vi "Write Config Data VI.vi"(8 "error in (no error)":errorcluster, 10 "Config Data":T1={"DS First Launch"=FALSE, "LogBaseFolder"=path "", "Live Logging"=FALSE, "Server Port"=0, "Max Number ML Rows"=0, "AM.WinBounds"={"Left"=0, "Top"=0, "Right"=0, "Bottom"=0}, "AM.FP.State"=enum."Invalid", "AM.Monitor"=0, "AM.Column Widths"=[], "ML.Visible Columns"=[], "ML.Splitter Position"=0, "ML.Column Widths"=[], "ML.WinBounds"={"Left"=0, "Top"=0, "Right"=0, "Bottom"=0}, "ML.FP.State"=enum."Invalid", "ML.Monitor"=0}, 11 "Settings in":refnum<class "Settings.lvclass">) -> (0 "error out":errorcluster, 3 "Settings out":refnum<class "Settings.lvclass">)   [LabVIEW 2017, in "Settings.lvclass"]
uses:
  Settings.lvclass
  Config Data.ctl
  <vilib>/Utility/miscctls.llb/LVRectTypeDef.ctl
  <vilib>/Utility/config.llb/Write Key (Boolean).vi
  <vilib>/Utility/config.llb/Write Key (Path).vi
  <vilib>/Utility/config.llb/Write Key (U32).vi
  <vilib>/Utility/config.llb/Write Key (String).vi
  <vilib>/Utility/config.llb/Write Key (I32).vi
  <vilib>/Utility/config.llb/NI_LVConfig.lvlib
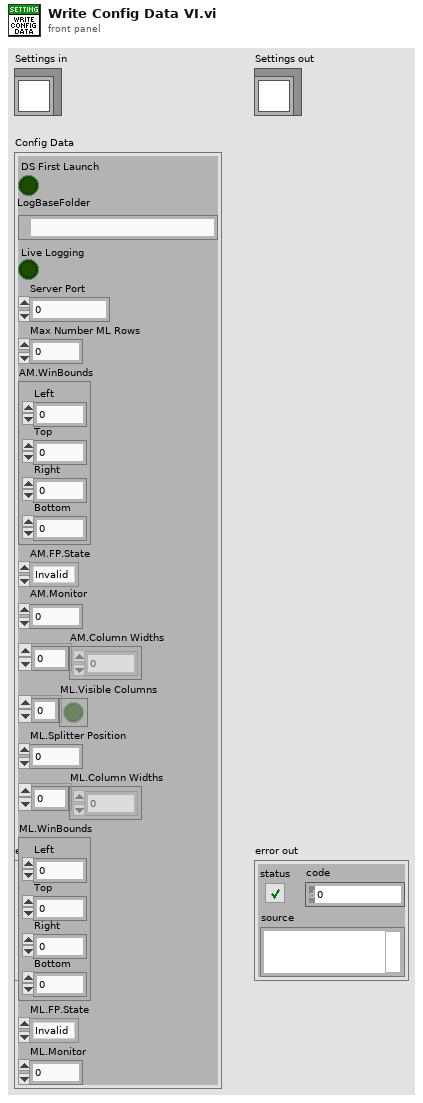
[diagram p1: front panel]
types:
  T1 = typedef "Settings.lvclass/Config Data.ctl" = cluster{"DS First Launch":bool, "LogBaseFolder":path, "Live Logging":bool, "Server Port":u16, "Max Number ML Rows":i32, "AM.WinBounds":T2, "AM.FP.State":enum32{"Invalid", "Standard", "Closed", "Hidden", "Minimized", "Maximized"}, "AM.Monitor":u16, "AM.Column Widths":u32[], "ML.Visible Columns":bool[], "ML.Splitter Position":i32, "ML.Column Widths":u32[], "ML.WinBounds":T2, "ML.FP.State":enum32{"Invalid", "Standard", "Closed", "Hidden", "Minimized", "Maximized"}, "ML.Monitor":u16}
  T2 = typedef "LVRectTypeDef.ctl" = cluster{"Left":i16, "Top":i16, "Right":i16, "Bottom":i16}
  T3 = enum32{"Invalid", "Standard", "Closed", "Hidden", "Minimized", "Maximized"}
  T4 = typedef "NI_LVConfig.lvlib/Config Data RefNum.ctl" = refnum<k1>
  T5 = typedef "LVAllMonitorsDisplayTypeDef.ctl" = cluster{"Bounds":cluster{"Left":i16, "Top":i16, "Right":i16, "Bottom":i16}, "Depth":i16}[]
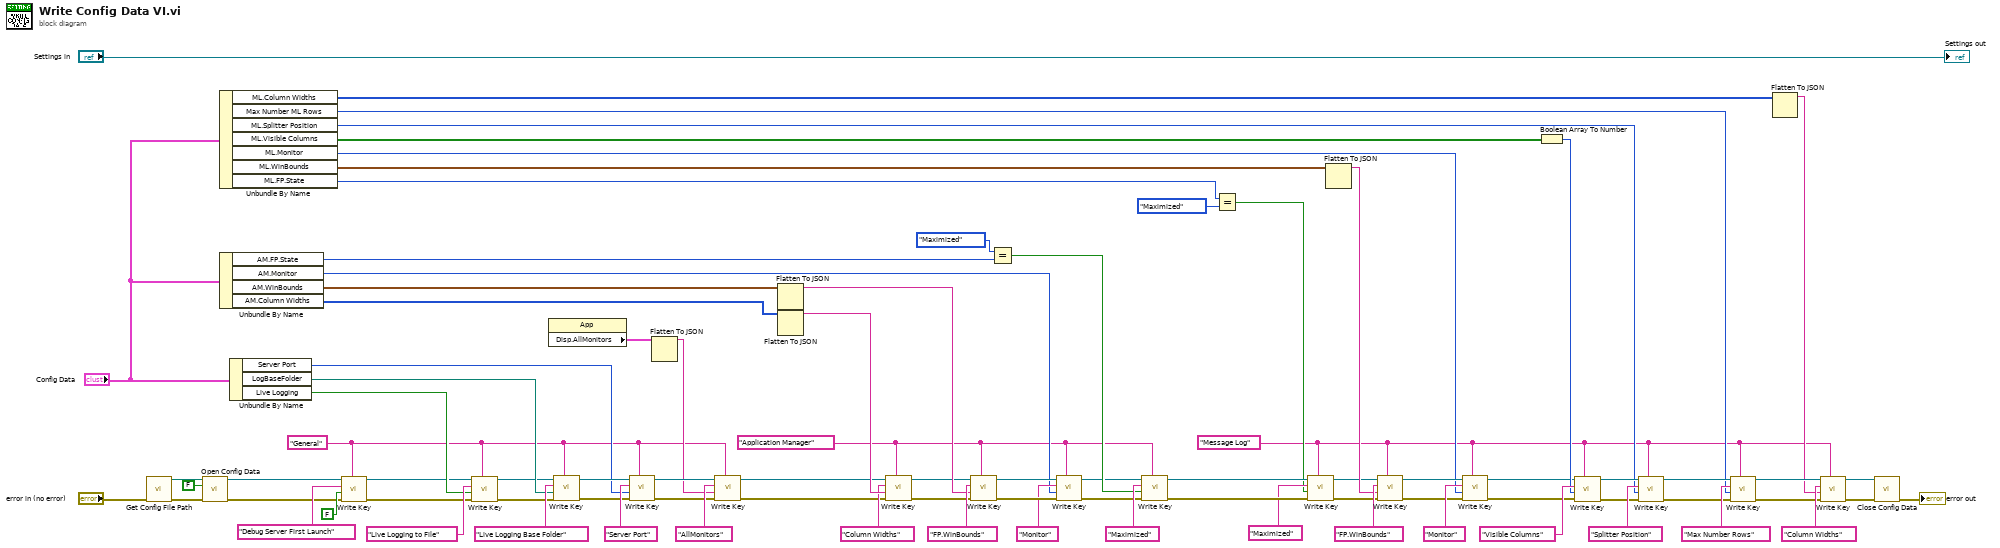
[diagram p0: block diagram]
diagram:
  w9 = "Message Log" ("section")
  w32 = "Application Manager" ("section")
  w1 = "General" ("section")
  n1 = call "Get Config File Path.vi"("error in (no error)"="error in (no error)") -> ("error out"=w71:errorcluster, "appended path"=w72:path)  [unwired: 9 in]
  n2 = call <vilib>:"Open Config Data.vi"("error in (no error)"=w71, "create file if necessary (T)"=FALSE, "configuration file path"=w72) -> ("error out"=w4:errorcluster, "refnum"=w5:T4)  [unwired: 6 in, 1 out]
  n3 = Unbundle By Name("Config Data") -> ("ML.Column Widths"=w37:u32[], "Max Number ML Rows"=w57:i32, "ML.Splitter Position"=w58:i32, "ML.Visible Columns"=w59:bool[], "ML.Monitor"=w23:u16, "ML.WinBounds"=w25:T2, "ML.FP.State"=w22:T3)
  n4 = Unbundle By Name("Config Data") -> ("AM.FP.State"=w56:T3, "AM.Monitor"=w49:u16, "AM.WinBounds"=w68:T2, "AM.Column Widths"=w40:u32[])
  n5 = Unbundle By Name("Config Data") -> ("Server Port"=w33:u16, "LogBaseFolder"=w74:path, "Live Logging"=w76:bool)
  n6 = call-poly <vilib>:"Write Key.vi"("section"=w1, "error in (no error)"=w4, "value"=FALSE ("default value"), "key"="Debug Server First Launch" ("name or relative path"), "refnum"=w5) -> ("error out"=w3:errorcluster, "refnum out"=w2:T4)  [unwired: 4 in, 1 out]
  n7 = call-poly <vilib>:"Write Key.vi"("section"=w1, "error in (no error)"=w3, "value"=w76, "key"="Live Logging to File", "refnum"=w2) -> ("error out"=w66:errorcluster, "refnum out"=w67:T4)  [unwired: 4 in, 1 out]
  n8 = property class="App"() -> ("Disp.AllMonitors"=w13:T5)  [unwired: 2 in, 2 out]
  n9 = call-poly <vilib>:"Write Key.vi"("section"=w1, "error in (no error)"=w66, "value"=w74, "key"="Live Logging Base Folder", "refnum"=w67) -> ("error out"=w35:errorcluster, "refnum out"=w34:T4)  [unwired: 4 in, 1 out]
  n10 = call-poly <vilib>:"Write Key.vi"("section"=w1, "error in (no error)"=w35, "value"=w33, "key"="Server Port", "refnum"=w34) -> ("error out"=w15:errorcluster, "refnum out"=w14:T4)  [unwired: 4 in, 1 out]
  n11 = Flatten To JSON(anything=w13) -> (JSON string=w12:string)  [unwired: 2 in, 1 out]
  n12 = call-poly <vilib>:"Write Key.vi"("section"=w1, "error in (no error)"=w15, "value"=w12, "key"="AllMonitors", "refnum"=w14) -> ("error out"=w11:errorcluster, "refnum out"=w10:T4)  [unwired: 4 in, 1 out]
  n13 = Flatten To JSON(anything=w68) -> (JSON string=w81:string)  [unwired: 2 in, 1 out]
  n14 = Flatten To JSON(anything=w40) -> (JSON string=w39:string)  [unwired: 2 in, 1 out]
  n15 = call-poly <vilib>:"Write Key.vi"("section"=w32, "error in (no error)"=w11, "value"=w39, "key"="Column Widths", "refnum"=w10) -> ("error out"=w42:errorcluster, "refnum out"=w41:T4)  [unwired: 4 in, 1 out]
  n16 = call-poly <vilib>:"Write Key.vi"("section"=w32, "error in (no error)"=w42, "value"=w81, "key"="FP.WinBounds", "refnum"=w41) -> ("error out"=w69:errorcluster, "refnum out"=w52:T4)  [unwired: 4 in, 1 out]
  n17 = Equal?(x=T3."Maximized" ("y"), y=w56) -> (x = y?=w78:bool)
  n18 = call-poly <vilib>:"Write Key.vi"("section"=w32, "error in (no error)"=w69, "value"=w49, "key"="Monitor", "refnum"=w52) -> ("error out"=w53:errorcluster, "refnum out"=w51:T4)  [unwired: 4 in, 1 out]
  n19 = call-poly <vilib>:"Write Key.vi"("section"=w32, "error in (no error)"=w53, "value"=w78, "key"="Maximized", "refnum"=w51) -> ("error out"=w55:errorcluster, "refnum out"=w54:T4)  [unwired: 4 in, 1 out]
  n20 = Equal?(x=w22, y=T3."Maximized") -> (x = y?=w17:bool)
  n21 = call-poly <vilib>:"Write Key.vi"("section"=w9, "error in (no error)"=w55, "value"=w17, "key"="Maximized", "refnum"=w54) -> ("error out"=w20:errorcluster, "refnum out"=w19:T4)  [unwired: 4 in, 1 out]
  n22 = Flatten To JSON(anything=w25) -> (JSON string=w24:string)  [unwired: 2 in, 1 out]
  n23 = call-poly <vilib>:"Write Key.vi"("section"=w9, "error in (no error)"=w20, "value"=w24, "key"="FP.WinBounds", "refnum"=w19) -> ("error out"=w27:errorcluster, "refnum out"=w29:T4)  [unwired: 4 in, 1 out]
  n24 = call-poly <vilib>:"Write Key.vi"("section"=w9, "error in (no error)"=w27, "value"=w23, "key"="Monitor", "refnum"=w29) -> ("error out"=w28:errorcluster, "refnum out"=w8:T4)  [unwired: 4 in, 1 out]
  n25 = Boolean Array To Number(Boolean array=w59) -> (number=w60:u32)
  n26 = call-poly <vilib>:"Write Key.vi"("section"=w9, "error in (no error)"=w28, "value"=w60, "key"="Visible Columns", "refnum"=w8) -> ("error out"=w61:errorcluster, "refnum out"=w62:T4)  [unwired: 4 in, 1 out]
  n27 = call-poly <vilib>:"Write Key.vi"("section"=w9, "error in (no error)"=w61, "value"=w58, "key"="Splitter Position", "refnum"=w62) -> ("error out"=w63:errorcluster, "refnum out"=w64:T4)  [unwired: 4 in, 1 out]
  n28 = call-poly <vilib>:"Write Key.vi"("section"=w9, "error in (no error)"=w63, "value"=w57, "key"="Max Number Rows", "refnum"=w64) -> ("error out"=w47:errorcluster, "refnum out"=w46:T4)  [unwired: 4 in, 1 out]
  n29 = Flatten To JSON(anything=w37) -> (JSON string=w43:string)  [unwired: 2 in, 1 out]
  n30 = call-poly <vilib>:"Write Key.vi"("section"=w9, "error in (no error)"=w47, "value"=w43, "key"="Column Widths", "refnum"=w46) -> ("error out"=w44:errorcluster, "refnum out"=w45:T4)  [unwired: 4 in, 1 out]
  n31 = call <vilib>:"Close Config Data.vi"("error in (no error)"=w44, "refnum"=w45) -> ("error out"=→"error out":errorcluster)  [unwired: 8 in, 1 out]
  "Settings out" <- "Settings in"
